vi "VariablesToString_Scalar.vi"(3 "Format":string="%0.2f", 4 "Terminate?":bool=TRUE, 5 "ValueIn":dbl, 6 "FieldName":string, 7 "Type":enum16{"Normal", "Matlab"}(ring)) -> (1 "StringOut":string)   [LabVIEW 2013]
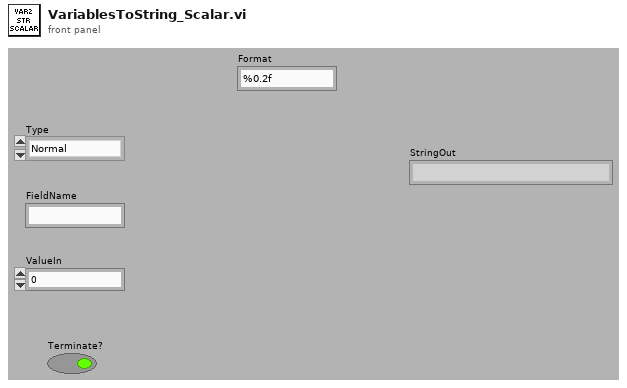
[diagram p1: front panel]
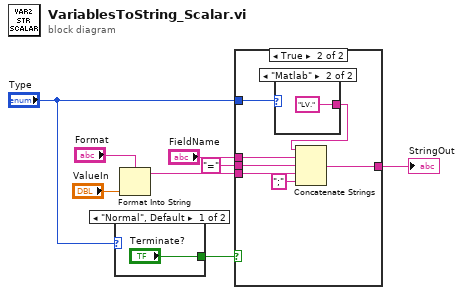
[diagram p0: block diagram]
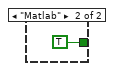
[diagram p2: hidden frame]
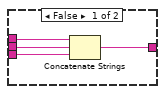
[diagram p3: hidden frame]
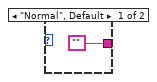
[diagram p4: hidden frame]
diagram:
  n1 = case shown="\"Normal\", Default" "Type" {
    tunnel: ["Terminate?" TRUE ("Terminate?")] -> w2
    frame "Normal", Default {
    }
    frame "Matlab" {
    }
  }
  n2 = Format Into String(format string="Format", "ValueIn") -> (resulting string=w4:string)  [unwired: 2 in, 1 out]
  n3 = case shown="True" w2 {
    tunnel: "FieldName" -> [w14 w21]
    tunnel: "=" ("string") -> [w13 w20]
    tunnel: [w12 w18] -> w6
    tunnel: w4 -> [w11 w17]
    tunnel: "Type" -> [_ w15]
    frame False {
      n4 = Concatenate Strings(w14, w13, w11) -> (w12:string)
    }
    frame True {
      n5 = case shown="\"Matlab\"" w15 {
        tunnel: ["" "LV."] -> w16
        frame "Normal", Default {
        }
        frame "Matlab" {
        }
      }
      n6 = Concatenate Strings(w16, w21, w20, w17, ";" ("string")) -> (w18:string)
    }
  }
  "StringOut" <- w6
